vi "LabVIEW Time to FPGA Time.vi"(1 "LabVIEW time":timestamp format="%<%.9X\n%x>T") -> (0 "FPGA time (ns)":u64)   [LabVIEW 2020, in "FPGA Timekeeper.lvlib"]
doc: "Converts LabVIEW Time into FPGA Time. Note that the FPGA Timekeeper keeps time in nanoseconds starting from January 1st, 1970."
uses:
  FPGA Timekeeper.lvlib
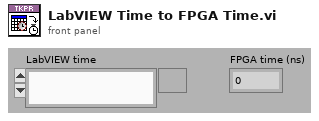
[diagram p1: front panel]
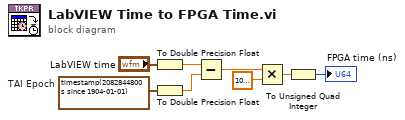
[diagram p0: block diagram]
diagram:
  w8 = timestamp(2082844800 s since 1904-01-01)  # TAI Epoch
  n1 = To Double Precision Float(number="LabVIEW time") -> (double precision float=w5:dbl)
  n2 = To Double Precision Float(number=w8) -> (double precision float=w4:dbl)
  n3 = Subtract(x=w5, y=w4) -> (x-y=w3:dbl)
  n4 = Multiply(x=w3, y=1000000000.0) -> (x*y=w2:dbl)
  n5 = To Unsigned Quad Integer(1:w2) -> (0:→"FPGA time (ns)":u64)
